vi "funnels to Commands.vi"(1 "funnels":T7(array[cluster]), 2 "Funnel Properties":T3[](array[typedef])=[{"Enabled"=TRUE, "Direction"=0, "Smooth Segments"=12.0, "Bottom Segs."=20.0, "Speed (um/s)"={"Schedule"=enum."Constant", "Settings"=variant(dbl 0.0)}, "Voltage (V)"={"Schedule"=enum."Constant", "Settings"=variant(dbl 0.0)}, "Set Resistance"=enum."1G ohm"}, {"Enabled"=TRUE, "Direction"=0, "Smooth Segments"=12.0, "Bottom Segs."=20.0, "Speed (um/s)"={"Schedule"=enum."Constant", "Settings"=variant(dbl 0.0)}, "Voltage (V)"={"Schedule"=enum."Constant", "Settings"=variant(dbl 0.0)}, "Set Resistance"=enum."1G ohm"}, {"Enabled"=TRUE, "Direction"=0, "Smooth Segments"=12.0, "Bottom Segs."=20.0, "Speed (um/s)"={"Schedule"=enum."Constant", "Settings"=variant(dbl 0.0)}, "Voltage (V)"={"Schedule"=enum."Constant", "Settings"=variant(dbl 0.0)}, "Set Resistance"=enum."1G ohm"}, {"Enabled"=TRUE, "Direction"=0, "Smooth Segments"=12.0, "Bottom Segs."=20.0, "Speed (um/s)"={"Schedule"=enum."Constant", "Settings"=variant(dbl 0.0)}, "Voltage (V)"={"Schedule"=enum."Constant", "Settings"=variant(dbl 0.0)}, "Set Resistance"=enum."1G ohm"}, {"Enabled"=TRUE, "Direction"=0, "Smooth Segments"=12.0, "Bottom Segs."=20.0, "Speed (um/s)"={"Schedule"=enum."Constant", "Settings"=variant(dbl 0.0)}, "Voltage (V)"={"Schedule"=enum."Constant", "Settings"=variant(dbl 0.0)}, "Set Resistance"=enum."1G ohm"}, {"Enabled"=TRUE, "Direction"=0, "Smooth Segments"=12.0, "Bottom Segs."=20.0, "Speed (um/s)"={"Schedule"=enum."Constant", "Settings"=variant(dbl 0.0)}, "Voltage (V)"={"Schedule"=enum."Constant", "Settings"=variant(dbl 0.0)}, "Set Resistance"=enum."1G ohm"}, {"Enabled"=TRUE, "Direction"=0, "Smooth Segments"=12.0, "Bottom Segs."=20.0, "Speed (um/s)"={"Schedule"=enum."Constant", "Settings"=variant(dbl 0.0)}, "Voltage (V)"={"Schedule"=enum."Constant", "Settings"=variant(dbl 0.0)}, "Set Resistance"=enum."1G ohm"}, {"Enabled"=TRUE, "Direction"=0, "Smooth Segments"=12.0, "Bottom Segs."=20.0, "Speed (um/s)"={"Schedule"=enum."Constant", "Settings"=variant(dbl 0.0)}, "Voltage (V)"={"Schedule"=enum."Constant", "Settings"=variant(dbl 0.0)}, "Set Resistance"=enum."1G ohm"}, {"Enabled"=TRUE, "Direction"=0, "Smooth Segments"=12.0, "Bottom Segs."=20.0, "Speed (um/s)"={"Schedule"=enum."Constant", "Settings"=variant(dbl 0.0)}, "Voltage (V)"={"Schedule"=enum."Constant", "Settings"=variant(dbl 0.0)}, "Set Resistance"=enum."1G ohm"}, {"Enabled"=TRUE, "Direction"=0, "Smooth Segments"=12.0, "Bottom Segs."=20.0, "Speed (um/s)"={"Schedule"=enum."Constant", "Settings"=variant(dbl 0.0)}, "Voltage (V)"={"Schedule"=enum."Constant", "Settings"=variant(dbl 0.0)}, "Set Resistance"=enum."1G ohm"}, {"Enabled"=TRUE, "Direction"=0, "Smooth Segments"=12.0, "Bottom Segs."=20.0, "Speed (um/s)"={"Schedule"=enum."Constant", "Settings"=variant(dbl 0.0)}, "Voltage (V)"={"Schedule"=enum."Constant", "Settings"=variant(dbl 0.0)}, "Set Resistance"=enum."1G ohm"}, {"Enabled"=TRUE, "Direction"=0, "Smooth Segments"=12.0, "Bottom Segs."=20.0, "Speed (um/s)"={"Schedule"=enum."Constant", "Settings"=variant(dbl 0.0)}, "Voltage (V)"={"Schedule"=enum."Constant", "Settings"=variant(dbl 0.0)}, "Set Resistance"=enum."1G ohm"}, {"Enabled"=TRUE, "Direction"=0, "Smooth Segments"=12.0, "Bottom Segs."=20.0, "Speed (um/s)"={"Schedule"=enum."Constant", "Settings"=variant(dbl 0.0)}, "Voltage (V)"={"Schedule"=enum."Constant", "Settings"=variant(dbl 0.0)}, "Set Resistance"=enum."1G ohm"}, {"Enabled"=TRUE, "Direction"=0, "Smooth Segments"=12.0, "Bottom Segs."=20.0, "Speed (um/s)"={"Schedule"=enum."Constant", "Settings"=variant(dbl 0.0)}, "Voltage (V)"={"Schedule"=enum."Constant", "Settings"=variant(dbl 0.0)}, "Set Resistance"=enum."1G ohm"}, {"Enabled"=TRUE, "Direction"=0, "Smooth Segments"=12.0, "Bottom Segs."=20.0, "Speed (um/s)"={"Schedule"=enum."Constant", "Settings"=variant(dbl 0.0)}, "Voltage (V)"={"Schedule"=enum."Constant", "Settings"=variant(dbl 0.0)}, "Set Resistance"=enum."1G ohm"}, {"Enabled"=TRUE, "Direction"=0, "Smooth Segments"=12.0, "Bottom Segs."=20.0, "Speed (um/s)"={"Schedule"=enum."Constant", "Settings"=variant(dbl 0.0)}, "Voltage (V)"={"Schedule"=enum."Constant", "Settings"=variant(dbl 0.0)}, "Set Resistance"=enum."1G ohm"}, {"Enabled"=TRUE, "Direction"=0, "Smooth Segments"=12.0, "Bottom Segs."=20.0, "Speed (um/s)"={"Schedule"=enum."Constant", "Settings"=variant(dbl 0.0)}, "Voltage (V)"={"Schedule"=enum."Constant", "Settings"=variant(dbl 0.0)}, "Set Resistance"=enum."1G ohm"}, {"Enabled"=TRUE, "Direction"=0, "Smooth Segments"=12.0, "Bottom Segs."=20.0, "Speed (um/s)"={"Schedule"=enum."Constant", "Settings"=variant(dbl 0.0)}, "Voltage (V)"={"Schedule"=enum."Constant", "Settings"=variant(dbl 0.0)}, "Set Resistance"=enum."1G ohm"}, {"Enabled"=TRUE, "Direction"=0, "Smooth Segments"=12.0, "Bottom Segs."=20.0, "Speed (um/s)"={"Schedule"=enum."Constant", "Settings"=variant(dbl 0.0)}, "Voltage (V)"={"Schedule"=enum."Constant", "Settings"=variant(dbl 0.0)}, "Set Resistance"=enum."1G ohm"}, {"Enabled"=TRUE, "Direction"=0, "Smooth Segments"=12.0, "Bottom Segs."=20.0, "Speed (um/s)"={"Schedule"=enum."Constant", "Settings"=variant(dbl 0.0)}, "Voltage (V)"={"Schedule"=enum."Constant", "Settings"=variant(dbl 0.0)}, "Set Resistance"=enum."1G ohm"}, {"Enabled"=TRUE, "Direction"=0, "Smooth Segments"=12.0, "Bottom Segs."=20.0, "Speed (um/s)"={"Schedule"=enum."Constant", "Settings"=variant(dbl 0.0)}, "Voltage (V)"={"Schedule"=enum."Constant", "Settings"=variant(dbl 0.0)}, "Set Resistance"=enum."1G ohm"}, {"Enabled"=TRUE, "Direction"=0, "Smooth Segments"=12.0, "Bottom Segs."=20.0, "Speed (um/s)"={"Schedule"=enum."Constant", "Settings"=variant(dbl 0.0)}, "Voltage (V)"={"Schedule"=enum."Constant", "Settings"=variant(dbl 0.0)}, "Set Resistance"=enum."1G ohm"}, {"Enabled"=TRUE, "Direction"=0, "Smooth Segments"=12.0, "Bottom Segs."=20.0, "Speed (um/s)"={"Schedule"=enum."Constant", "Settings"=variant(dbl 0.0)}, "Voltage (V)"={"Schedule"=enum."Constant", "Settings"=variant(dbl 0.0)}, "Set Resistance"=enum."1G ohm"}, {"Enabled"=TRUE, "Direction"=0, "Smooth Segments"=12.0, "Bottom Segs."=20.0, "Speed (um/s)"={"Schedule"=enum."Constant", "Settings"=variant(dbl 0.0)}, "Voltage (V)"={"Schedule"=enum."Constant", "Settings"=variant(dbl 0.0)}, "Set Resistance"=enum."1G ohm"}, {"Enabled"=TRUE, "Direction"=0, "Smooth Segments"=12.0, "Bottom Segs."=20.0, "Speed (um/s)"={"Schedule"=enum."Constant", "Settings"=variant(dbl 0.0)}, "Voltage (V)"={"Schedule"=enum."Constant", "Settings"=variant(dbl 0.0)}, "Set Resistance"=enum."1G ohm"}, {"Enabled"=TRUE, "Direction"=0, "Smooth Segments"=12.0, "Bottom Segs."=20.0, "Speed (um/s)"={"Schedule"=enum."Constant", "Settings"=variant(dbl 0.0)}, "Voltage (V)"={"Schedule"=enum."Constant", "Settings"=variant(dbl 0.0)}, "Set Resistance"=enum."1G ohm"}, {"Enabled"=TRUE, "Direction"=0, "Smooth Segments"=12.0, "Bottom Segs."=20.0, "Speed (um/s)"={"Schedule"=enum."Constant", "Settings"=variant(dbl 0.0)}, "Voltage (V)"={"Schedule"=enum."Constant", "Settings"=variant(dbl 0.0)}, "Set Resistance"=enum."1G ohm"}, {"Enabled"=TRUE, "Direction"=0, "Smooth Segments"=12.0, "Bottom Segs."=20.0, "Speed (um/s)"={"Schedule"=enum."Constant", "Settings"=variant(dbl 0.0)}, "Voltage (V)"={"Schedule"=enum."Constant", "Settings"=variant(dbl 0.0)}, "Set Resistance"=enum."1G ohm"}, {"Enabled"=TRUE, "Direction"=0, "Smooth Segments"=12.0, "Bottom Segs."=20.0, "Speed (um/s)"={"Schedule"=enum."Constant", "Settings"=variant(dbl 0.0)}, "Voltage (V)"={"Schedule"=enum."Constant", "Settings"=variant(dbl 0.0)}, "Set Resistance"=enum."1G ohm"}, {"Enabled"=TRUE, "Direction"=0, "Smooth Segments"=12.0, "Bottom Segs."=20.0, "Speed (um/s)"={"Schedule"=enum."Constant", "Settings"=variant(dbl 0.0)}, "Voltage (V)"={"Schedule"=enum."Constant", "Settings"=variant(dbl 0.0)}, "Set Resistance"=enum."1G ohm"}, {"Enabled"=TRUE, "Direction"=0, "Smooth Segments"=12.0, "Bottom Segs."=20.0, "Speed (um/s)"={"Schedule"=enum."Constant", "Settings"=variant(dbl 0.0)}, "Voltage (V)"={"Schedule"=enum."Constant", "Settings"=variant(dbl 0.0)}, "Set Resistance"=enum."1G ohm"}, {"Enabled"=TRUE, "Direction"=0, "Smooth Segments"=12.0, "Bottom Segs."=20.0, "Speed (um/s)"={"Schedule"=enum."Constant", "Settings"=variant(dbl 0.0)}, "Voltage (V)"={"Schedule"=enum."Constant", "Settings"=variant(dbl 0.0)}, "Set Resistance"=enum."1G ohm"}, {"Enabled"=TRUE, "Direction"=0, "Smooth Segments"=12.0, "Bottom Segs."=20.0, "Speed (um/s)"={"Schedule"=enum."Constant", "Settings"=variant(dbl 0.0)}, "Voltage (V)"={"Schedule"=enum."Constant", "Settings"=variant(dbl 0.0)}, "Set Resistance"=enum."1G ohm"}, {"Enabled"=TRUE, "Direction"=0, "Smooth Segments"=12.0, "Bottom Segs."=20.0, "Speed (um/s)"={"Schedule"=enum."Constant", "Settings"=variant(dbl 0.0)}, "Voltage (V)"={"Schedule"=enum."Constant", "Settings"=variant(dbl 0.0)}, "Set Resistance"=enum."1G ohm"}, {"Enabled"=TRUE, "Direction"=0, "Smooth Segments"=12.0, "Bottom Segs."=20.0, "Speed (um/s)"={"Schedule"=enum."Constant", "Settings"=variant(dbl 0.0)}, "Voltage (V)"={"Schedule"=enum."Constant", "Settings"=variant(dbl 0.0)}, "Set Resistance"=enum."1G ohm"}, {"Enabled"=TRUE, "Direction"=0, "Smooth Segments"=12.0, "Bottom Segs."=20.0, "Speed (um/s)"={"Schedule"=enum."Constant", "Settings"=variant(dbl 0.0)}, "Voltage (V)"={"Schedule"=enum."Constant", "Settings"=variant(dbl 0.0)}, "Set Resistance"=enum."1G ohm"}, {"Enabled"=TRUE, "Direction"=0, "Smooth Segments"=12.0, "Bottom Segs."=20.0, "Speed (um/s)"={"Schedule"=enum."Constant", "Settings"=variant(dbl 0.0)}, "Voltage (V)"={"Schedule"=enum."Constant", "Settings"=variant(dbl 0.0)}, "Set Resistance"=enum."1G ohm"}, {"Enabled"=TRUE, "Direction"=0, "Smooth Segments"=12.0, "Bottom Segs."=20.0, "Speed (um/s)"={"Schedule"=enum."Constant", "Settings"=variant(dbl 0.0)}, "Voltage (V)"={"Schedule"=enum."Constant", "Settings"=variant(dbl 0.0)}, "Set Resistance"=enum."1G ohm"}, {"Enabled"=TRUE, "Direction"=0, "Smooth Segments"=12.0, "Bottom Segs."=20.0, "Speed (um/s)"={"Schedule"=enum."Constant", "Settings"=variant(dbl 0.0)}, "Voltage (V)"={"Schedule"=enum."Constant", "Settings"=variant(dbl 0.0)}, "Set Resistance"=enum."1G ohm"}, {"Enabled"=TRUE, "Direction"=0, "Smooth Segments"=12.0, "Bottom Segs."=20.0, "Speed (um/s)"={"Schedule"=enum."Constant", "Settings"=variant(dbl 0.0)}, "Voltage (V)"={"Schedule"=enum."Constant", "Settings"=variant(dbl 0.0)}, "Set Resistance"=enum."1G ohm"}, {"Enabled"=TRUE, "Direction"=0, "Smooth Segments"=12.0, "Bottom Segs."=20.0, "Speed (um/s)"={"Schedule"=enum."Constant", "Settings"=variant(dbl 0.0)}, "Voltage (V)"={"Schedule"=enum."Constant", "Settings"=variant(dbl 0.0)}, "Set Resistance"=enum."1G ohm"}, {"Enabled"=TRUE, "Direction"=0, "Smooth Segments"=12.0, "Bottom Segs."=20.0, "Speed (um/s)"={"Schedule"=enum."Constant", "Settings"=variant(dbl 0.0)}, "Voltage (V)"={"Schedule"=enum."Constant", "Settings"=variant(dbl 0.0)}, "Set Resistance"=enum."1G ohm"}, {"Enabled"=TRUE, "Direction"=0, "Smooth Segments"=12.0, "Bottom Segs."=20.0, "Speed (um/s)"={"Schedule"=enum."Constant", "Settings"=variant(dbl 0.0)}, "Voltage (V)"={"Schedule"=enum."Constant", "Settings"=variant(dbl 0.0)}, "Set Resistance"=enum."1G ohm"}, {"Enabled"=TRUE, "Direction"=0, "Smooth Segments"=12.0, "Bottom Segs."=20.0, "Speed (um/s)"={"Schedule"=enum."Constant", "Settings"=variant(dbl 0.0)}, "Voltage (V)"={"Schedule"=enum."Constant", "Settings"=variant(dbl 0.0)}, "Set Resistance"=enum."1G ohm"}, {"Enabled"=TRUE, "Direction"=0, "Smooth Segments"=12.0, "Bottom Segs."=20.0, "Speed (um/s)"={"Schedule"=enum."Constant", "Settings"=variant(dbl 0.0)}, "Voltage (V)"={"Schedule"=enum."Constant", "Settings"=variant(dbl 0.0)}, "Set Resistance"=enum."1G ohm"}, {"Enabled"=TRUE, "Direction"=0, "Smooth Segments"=12.0, "Bottom Segs."=20.0, "Speed (um/s)"={"Schedule"=enum."Constant", "Settings"=variant(dbl 0.0)}, "Voltage (V)"={"Schedule"=enum."Constant", "Settings"=variant(dbl 0.0)}, "Set Resistance"=enum."1G ohm"}, {"Enabled"=TRUE, "Direction"=0, "Smooth Segments"=12.0, "Bottom Segs."=20.0, "Speed (um/s)"={"Schedule"=enum."Constant", "Settings"=variant(dbl 0.0)}, "Voltage (V)"={"Schedule"=enum."Constant", "Settings"=variant(dbl 0.0)}, "Set Resistance"=enum."1G ohm"}, {"Enabled"=TRUE, "Direction"=0, "Smooth Segments"=12.0, "Bottom Segs."=20.0, "Speed (um/s)"={"Schedule"=enum."Constant", "Settings"=variant(dbl 0.0)}, "Voltage (V)"={"Schedule"=enum."Constant", "Settings"=variant(dbl 0.0)}, "Set Resistance"=enum."1G ohm"}, {"Enabled"=TRUE, "Direction"=0, "Smooth Segments"=12.0, "Bottom Segs."=20.0, "Speed (um/s)"={"Schedule"=enum."Constant", "Settings"=variant(dbl 0.0)}, "Voltage (V)"={"Schedule"=enum."Constant", "Settings"=variant(dbl 0.0)}, "Set Resistance"=enum."1G ohm"}, {"Enabled"=TRUE, "Direction"=0, "Smooth Segments"=12.0, "Bottom Segs."=20.0, "Speed (um/s)"={"Schedule"=enum."Constant", "Settings"=variant(dbl 0.0)}, "Voltage (V)"={"Schedule"=enum."Constant", "Settings"=variant(dbl 0.0)}, "Set Resistance"=enum."1G ohm"}, {"Enabled"=TRUE, "Direction"=0, "Smooth Segments"=12.0, "Bottom Segs."=20.0, "Speed (um/s)"={"Schedule"=enum."Constant", "Settings"=variant(dbl 0.0)}, "Voltage (V)"={"Schedule"=enum."Constant", "Settings"=variant(dbl 0.0)}, "Set Resistance"=enum."1G ohm"}, {"Enabled"=TRUE, "Direction"=0, "Smooth Segments"=12.0, "Bottom Segs."=20.0, "Speed (um/s)"={"Schedule"=enum."Constant", "Settings"=variant(dbl 0.0)}, "Voltage (V)"={"Schedule"=enum."Constant", "Settings"=variant(dbl 0.0)}, "Set Resistance"=enum."1G ohm"}, {"Enabled"=TRUE, "Direction"=0, "Smooth Segments"=12.0, "Bottom Segs."=20.0, "Speed (um/s)"={"Schedule"=enum."Constant", "Settings"=variant(dbl 0.0)}, "Voltage (V)"={"Schedule"=enum."Constant", "Settings"=variant(dbl 0.0)}, "Set Resistance"=enum."1G ohm"}, {"Enabled"=TRUE, "Direction"=0, "Smooth Segments"=12.0, "Bottom Segs."=20.0, "Speed (um/s)"={"Schedule"=enum."Constant", "Settings"=variant(dbl 0.0)}, "Voltage (V)"={"Schedule"=enum."Constant", "Settings"=variant(dbl 0.0)}, "Set Resistance"=enum."1G ohm"}, {"Enabled"=TRUE, "Direction"=0, "Smooth Segments"=12.0, "Bottom Segs."=20.0, "Speed (um/s)"={"Schedule"=enum."Constant", "Settings"=variant(dbl 0.0)}, "Voltage (V)"={"Schedule"=enum."Constant", "Settings"=variant(dbl 0.0)}, "Set Resistance"=enum."1G ohm"}, {"Enabled"=TRUE, "Direction"=0, "Smooth Segments"=12.0, "Bottom Segs."=20.0, "Speed (um/s)"={"Schedule"=enum."Constant", "Settings"=variant(dbl 0.0)}, "Voltage (V)"={"Schedule"=enum."Constant", "Settings"=variant(dbl 0.0)}, "Set Resistance"=enum."1G ohm"}, {"Enabled"=TRUE, "Direction"=0, "Smooth Segments"=12.0, "Bottom Segs."=20.0, "Speed (um/s)"={"Schedule"=enum."Constant", "Settings"=variant(dbl 0.0)}, "Voltage (V)"={"Schedule"=enum."Constant", "Settings"=variant(dbl 0.0)}, "Set Resistance"=enum."1G ohm"}, {"Enabled"=TRUE, "Direction"=0, "Smooth Segments"=12.0, "Bottom Segs."=20.0, "Speed (um/s)"={"Schedule"=enum."Constant", "Settings"=variant(dbl 0.0)}, "Voltage (V)"={"Schedule"=enum."Constant", "Settings"=variant(dbl 0.0)}, "Set Resistance"=enum."1G ohm"}, {"Enabled"=TRUE, "Direction"=0, "Smooth Segments"=12.0, "Bottom Segs."=20.0, "Speed (um/s)"={"Schedule"=enum."Constant", "Settings"=variant(dbl 0.0)}, "Voltage (V)"={"Schedule"=enum."Constant", "Settings"=variant(dbl 0.0)}, "Set Resistance"=enum."1G ohm"}, {"Enabled"=TRUE, "Direction"=0, "Smooth Segments"=12.0, "Bottom Segs."=20.0, "Speed (um/s)"={"Schedule"=enum."Constant", "Settings"=variant(dbl 0.0)}, "Voltage (V)"={"Schedule"=enum."Constant", "Settings"=variant(dbl 0.0)}, "Set Resistance"=enum."1G ohm"}, {"Enabled"=TRUE, "Direction"=0, "Smooth Segments"=12.0, "Bottom Segs."=20.0, "Speed (um/s)"={"Schedule"=enum."Constant", "Settings"=variant(dbl 0.0)}, "Voltage (V)"={"Schedule"=enum."Constant", "Settings"=variant(dbl 0.0)}, "Set Resistance"=enum."1G ohm"}, {"Enabled"=TRUE, "Direction"=0, "Smooth Segments"=12.0, "Bottom Segs."=20.0, "Speed (um/s)"={"Schedule"=enum."Constant", "Settings"=variant(dbl 0.0)}, "Voltage (V)"={"Schedule"=enum."Constant", "Settings"=variant(dbl 0.0)}, "Set Resistance"=enum."1G ohm"}, {"Enabled"=TRUE, "Direction"=0, "Smooth Segments"=12.0, "Bottom Segs."=20.0, "Speed (um/s)"={"Schedule"=enum."Constant", "Settings"=variant(dbl 0.0)}, "Voltage (V)"={"Schedule"=enum."Constant", "Settings"=variant(dbl 0.0)}, "Set Resistance"=enum."1G ohm"}, {"Enabled"=TRUE, "Direction"=0, "Smooth Segments"=12.0, "Bottom Segs."=20.0, "Speed (um/s)"={"Schedule"=enum."Constant", "Settings"=variant(dbl 0.0)}, "Voltage (V)"={"Schedule"=enum."Constant", "Settings"=variant(dbl 0.0)}, "Set Resistance"=enum."1G ohm"}, {"Enabled"=TRUE, "Direction"=0, "Smooth Segments"=12.0, "Bottom Segs."=20.0, "Speed (um/s)"={"Schedule"=enum."Constant", "Settings"=variant(dbl 0.0)}, "Voltage (V)"={"Schedule"=enum."Constant", "Settings"=variant(dbl 0.0)}, "Set Resistance"=enum."1G ohm"}, {"Enabled"=TRUE, "Direction"=0, "Smooth Segments"=12.0, "Bottom Segs."=20.0, "Speed (um/s)"={"Schedule"=enum."Constant", "Settings"=variant(dbl 0.0)}, "Voltage (V)"={"Schedule"=enum."Constant", "Settings"=variant(dbl 0.0)}, "Set Resistance"=enum."1G ohm"}, {"Enabled"=TRUE, "Direction"=0, "Smooth Segments"=12.0, "Bottom Segs."=20.0, "Speed (um/s)"={"Schedule"=enum."Constant", "Settings"=variant(dbl 0.0)}, "Voltage (V)"={"Schedule"=enum."Constant", "Settings"=variant(dbl 0.0)}, "Set Resistance"=enum."1G ohm"}, {"Enabled"=TRUE, "Direction"=0, "Smooth Segments"=12.0, "Bottom Segs."=20.0, "Speed (um/s)"={"Schedule"=enum."Constant", "Settings"=variant(dbl 0.0)}, "Voltage (V)"={"Schedule"=enum."Constant", "Settings"=variant(dbl 0.0)}, "Set Resistance"=enum."1G ohm"}, {"Enabled"=TRUE, "Direction"=0, "Smooth Segments"=12.0, "Bottom Segs."=20.0, "Speed (um/s)"={"Schedule"=enum."Constant", "Settings"=variant(dbl 0.0)}, "Voltage (V)"={"Schedule"=enum."Constant", "Settings"=variant(dbl 0.0)}, "Set Resistance"=enum."1G ohm"}, {"Enabled"=TRUE, "Direction"=0, "Smooth Segments"=12.0, "Bottom Segs."=20.0, "Speed (um/s)"={"Schedule"=enum."Constant", "Settings"=variant(dbl 0.0)}, "Voltage (V)"={"Schedule"=enum."Constant", "Settings"=variant(dbl 0.0)}, "Set Resistance"=enum."1G ohm"}, {"Enabled"=TRUE, "Direction"=0, "Smooth Segments"=12.0, "Bottom Segs."=20.0, "Speed (um/s)"={"Schedule"=enum."Constant", "Settings"=variant(dbl 0.0)}, "Voltage (V)"={"Schedule"=enum."Constant", "Settings"=variant(dbl 0.0)}, "Set Resistance"=enum."1G ohm"}, {"Enabled"=TRUE, "Direction"=0, "Smooth Segments"=12.0, "Bottom Segs."=20.0, "Speed (um/s)"={"Schedule"=enum."Constant", "Settings"=variant(dbl 0.0)}, "Voltage (V)"={"Schedule"=enum."Constant", "Settings"=variant(dbl 0.0)}, "Set Resistance"=enum."1G ohm"}, {"Enabled"=TRUE, "Direction"=0, "Smooth Segments"=12.0, "Bottom Segs."=20.0, "Speed (um/s)"={"Schedule"=enum."Constant", "Settings"=variant(dbl 0.0)}, "Voltage (V)"={"Schedule"=enum."Constant", "Settings"=variant(dbl 0.0)}, "Set Resistance"=enum."1G ohm"}, {"Enabled"=TRUE, "Direction"=0, "Smooth Segments"=12.0, "Bottom Segs."=20.0, "Speed (um/s)"={"Schedule"=enum."Constant", "Settings"=variant(dbl 0.0)}, "Voltage (V)"={"Schedule"=enum."Constant", "Settings"=variant(dbl 0.0)}, "Set Resistance"=enum."1G ohm"}, {"Enabled"=TRUE, "Direction"=0, "Smooth Segments"=12.0, "Bottom Segs."=20.0, "Speed (um/s)"={"Schedule"=enum."Constant", "Settings"=variant(dbl 0.0)}, "Voltage (V)"={"Schedule"=enum."Constant", "Settings"=variant(dbl 0.0)}, "Set Resistance"=enum."1G ohm"}, {"Enabled"=TRUE, "Direction"=0, "Smooth Segments"=12.0, "Bottom Segs."=20.0, "Speed (um/s)"={"Schedule"=enum."Constant", "Settings"=variant(dbl 0.0)}, "Voltage (V)"={"Schedule"=enum."Constant", "Settings"=variant(dbl 0.0)}, "Set Resistance"=enum."1G ohm"}, {"Enabled"=TRUE, "Direction"=0, "Smooth Segments"=12.0, "Bottom Segs."=20.0, "Speed (um/s)"={"Schedule"=enum."Constant", "Settings"=variant(dbl 0.0)}, "Voltage (V)"={"Schedule"=enum."Constant", "Settings"=variant(dbl 0.0)}, "Set Resistance"=enum."1G ohm"}, {"Enabled"=TRUE, "Direction"=0, "Smooth Segments"=12.0, "Bottom Segs."=20.0, "Speed (um/s)"={"Schedule"=enum."Constant", "Settings"=variant(dbl 0.0)}, "Voltage (V)"={"Schedule"=enum."Constant", "Settings"=variant(dbl 0.0)}, "Set Resistance"=enum."1G ohm"}, {"Enabled"=TRUE, "Direction"=0, "Smooth Segments"=12.0, "Bottom Segs."=20.0, "Speed (um/s)"={"Schedule"=enum."Constant", "Settings"=variant(dbl 0.0)}, "Voltage (V)"={"Schedule"=enum."Constant", "Settings"=variant(dbl 0.0)}, "Set Resistance"=enum."1G ohm"}, {"Enabled"=TRUE, "Direction"=0, "Smooth Segments"=12.0, "Bottom Segs."=20.0, "Speed (um/s)"={"Schedule"=enum."Constant", "Settings"=variant(dbl 0.0)}, "Voltage (V)"={"Schedule"=enum."Constant", "Settings"=variant(dbl 0.0)}, "Set Resistance"=enum."1G ohm"}, {"Enabled"=TRUE, "Direction"=0, "Smooth Segments"=12.0, "Bottom Segs."=20.0, "Speed (um/s)"={"Schedule"=enum."Constant", "Settings"=variant(dbl 0.0)}, "Voltage (V)"={"Schedule"=enum."Constant", "Settings"=variant(dbl 0.0)}, "Set Resistance"=enum."1G ohm"}, {"Enabled"=TRUE, "Direction"=0, "Smooth Segments"=12.0, "Bottom Segs."=20.0, "Speed (um/s)"={"Schedule"=enum."Constant", "Settings"=variant(dbl 0.0)}, "Voltage (V)"={"Schedule"=enum."Constant", "Settings"=variant(dbl 0.0)}, "Set Resistance"=enum."1G ohm"}, {"Enabled"=TRUE, "Direction"=0, "Smooth Segments"=12.0, "Bottom Segs."=20.0, "Speed (um/s)"={"Schedule"=enum."Constant", "Settings"=variant(dbl 0.0)}, "Voltage (V)"={"Schedule"=enum."Constant", "Settings"=variant(dbl 0.0)}, "Set Resistance"=enum."1G ohm"}, {"Enabled"=TRUE, "Direction"=0, "Smooth Segments"=12.0, "Bottom Segs."=20.0, "Speed (um/s)"={"Schedule"=enum."Constant", "Settings"=variant(dbl 0.0)}, "Voltage (V)"={"Schedule"=enum."Constant", "Settings"=variant(dbl 0.0)}, "Set Resistance"=enum."1G ohm"}, {"Enabled"=TRUE, "Direction"=0, "Smooth Segments"=12.0, "Bottom Segs."=20.0, "Speed (um/s)"={"Schedule"=enum."Constant", "Settings"=variant(dbl 0.0)}, "Voltage (V)"={"Schedule"=enum."Constant", "Settings"=variant(dbl 0.0)}, "Set Resistance"=enum."1G ohm"}, {"Enabled"=TRUE, "Direction"=0, "Smooth Segments"=12.0, "Bottom Segs."=20.0, "Speed (um/s)"={"Schedule"=enum."Constant", "Settings"=variant(dbl 0.0)}, "Voltage (V)"={"Schedule"=enum."Constant", "Settings"=variant(dbl 0.0)}, "Set Resistance"=enum."1G ohm"}, {"Enabled"=TRUE, "Direction"=0, "Smooth Segments"=12.0, "Bottom Segs."=20.0, "Speed (um/s)"={"Schedule"=enum."Constant", "Settings"=variant(dbl 0.0)}, "Voltage (V)"={"Schedule"=enum."Constant", "Settings"=variant(dbl 0.0)}, "Set Resistance"=enum."1G ohm"}, {"Enabled"=TRUE, "Direction"=0, "Smooth Segments"=12.0, "Bottom Segs."=20.0, "Speed (um/s)"={"Schedule"=enum."Constant", "Settings"=variant(dbl 0.0)}, "Voltage (V)"={"Schedule"=enum."Constant", "Settings"=variant(dbl 0.0)}, "Set Resistance"=enum."1G ohm"}, {"Enabled"=TRUE, "Direction"=0, "Smooth Segments"=12.0, "Bottom Segs."=20.0, "Speed (um/s)"={"Schedule"=enum."Constant", "Settings"=variant(dbl 0.0)}, "Voltage (V)"={"Schedule"=enum."Constant", "Settings"=variant(dbl 0.0)}, "Set Resistance"=enum."1G ohm"}, {"Enabled"=TRUE, "Direction"=0, "Smooth Segments"=12.0, "Bottom Segs."=20.0, "Speed (um/s)"={"Schedule"=enum."Constant", "Settings"=variant(dbl 0.0)}, "Voltage (V)"={"Schedule"=enum."Constant", "Settings"=variant(dbl 0.0)}, "Set Resistance"=enum."1G ohm"}, {"Enabled"=TRUE, "Direction"=0, "Smooth Segments"=12.0, "Bottom Segs."=20.0, "Speed (um/s)"={"Schedule"=enum."Constant", "Settings"=variant(dbl 0.0)}, "Voltage (V)"={"Schedule"=enum."Constant", "Settings"=variant(dbl 0.0)}, "Set Resistance"=enum."1G ohm"}, {"Enabled"=TRUE, "Direction"=0, "Smooth Segments"=12.0, "Bottom Segs."=20.0, "Speed (um/s)"={"Schedule"=enum."Constant", "Settings"=variant(dbl 0.0)}, "Voltage (V)"={"Schedule"=enum."Constant", "Settings"=variant(dbl 0.0)}, "Set Resistance"=enum."1G ohm"}, {"Enabled"=TRUE, "Direction"=0, "Smooth Segments"=12.0, "Bottom Segs."=20.0, "Speed (um/s)"={"Schedule"=enum."Constant", "Settings"=variant(dbl 0.0)}, "Voltage (V)"={"Schedule"=enum."Constant", "Settings"=variant(dbl 0.0)}, "Set Resistance"=enum."1G ohm"}, {"Enabled"=TRUE, "Direction"=0, "Smooth Segments"=12.0, "Bottom Segs."=20.0, "Speed (um/s)"={"Schedule"=enum."Constant", "Settings"=variant(dbl 0.0)}, "Voltage (V)"={"Schedule"=enum."Constant", "Settings"=variant(dbl 0.0)}, "Set Resistance"=enum."1G ohm"}, {"Enabled"=TRUE, "Direction"=0, "Smooth Segments"=12.0, "Bottom Segs."=20.0, "Speed (um/s)"={"Schedule"=enum."Constant", "Settings"=variant(dbl 0.0)}, "Voltage (V)"={"Schedule"=enum."Constant", "Settings"=variant(dbl 0.0)}, "Set Resistance"=enum."1G ohm"}, {"Enabled"=TRUE, "Direction"=0, "Smooth Segments"=12.0, "Bottom Segs."=20.0, "Speed (um/s)"={"Schedule"=enum."Constant", "Settings"=variant(dbl 0.0)}, "Voltage (V)"={"Schedule"=enum."Constant", "Settings"=variant(dbl 0.0)}, "Set Resistance"=enum."1G ohm"}, {"Enabled"=TRUE, "Direction"=0, "Smooth Segments"=12.0, "Bottom Segs."=20.0, "Speed (um/s)"={"Schedule"=enum."Constant", "Settings"=variant(dbl 0.0)}, "Voltage (V)"={"Schedule"=enum."Constant", "Settings"=variant(dbl 0.0)}, "Set Resistance"=enum."1G ohm"}, {"Enabled"=TRUE, "Direction"=0, "Smooth Segments"=12.0, "Bottom Segs."=20.0, "Speed (um/s)"={"Schedule"=enum."Constant", "Settings"=variant(dbl 0.0)}, "Voltage (V)"={"Schedule"=enum."Constant", "Settings"=variant(dbl 0.0)}, "Set Resistance"=enum."1G ohm"}, {"Enabled"=TRUE, "Direction"=0, "Smooth Segments"=12.0, "Bottom Segs."=20.0, "Speed (um/s)"={"Schedule"=enum."Constant", "Settings"=variant(dbl 0.0)}, "Voltage (V)"={"Schedule"=enum."Constant", "Settings"=variant(dbl 0.0)}, "Set Resistance"=enum."1G ohm"}, {"Enabled"=TRUE, "Direction"=0, "Smooth Segments"=12.0, "Bottom Segs."=20.0, "Speed (um/s)"={"Schedule"=enum."Constant", "Settings"=variant(dbl 0.0)}, "Voltage (V)"={"Schedule"=enum."Constant", "Settings"=variant(dbl 0.0)}, "Set Resistance"=enum."1G ohm"}, {"Enabled"=TRUE, "Direction"=0, "Smooth Segments"=12.0, "Bottom Segs."=20.0, "Speed (um/s)"={"Schedule"=enum."Constant", "Settings"=variant(dbl 0.0)}, "Voltage (V)"={"Schedule"=enum."Constant", "Settings"=variant(dbl 0.0)}, "Set Resistance"=enum."1G ohm"}] {"Direction" items=["Forward", "Backward"]}) -> (0 "Lithography Data":T2(array[cluster]))   [LabVIEW 2019]
doc: "This VI processes the rectangles' data and outputs lithography data."
uses:
  <vilib>/Analysis/Matrix/Datatypes/RealMatrix.ctl
  typedefs/Funnel Properties - cluster.ctl
  typedefs/Voltage - cluster.ctl
  typedefs/Schedule - enum.ctl
  <userlib>/LevyLab/Relay Box/Typedefs/Resistor--enum.ctl
  <userlib>/_OpenG.lib/array/array.llb/Search 1D Array (String)__ogtk.vi
  <userlib>/LevyLab/Relay Box/Relay-Box.lvclass
  <vilib>/Analysis/Matrix/NI_Matrix.lvlib
panel:
  # "MONSTER CLUSTER!!!"
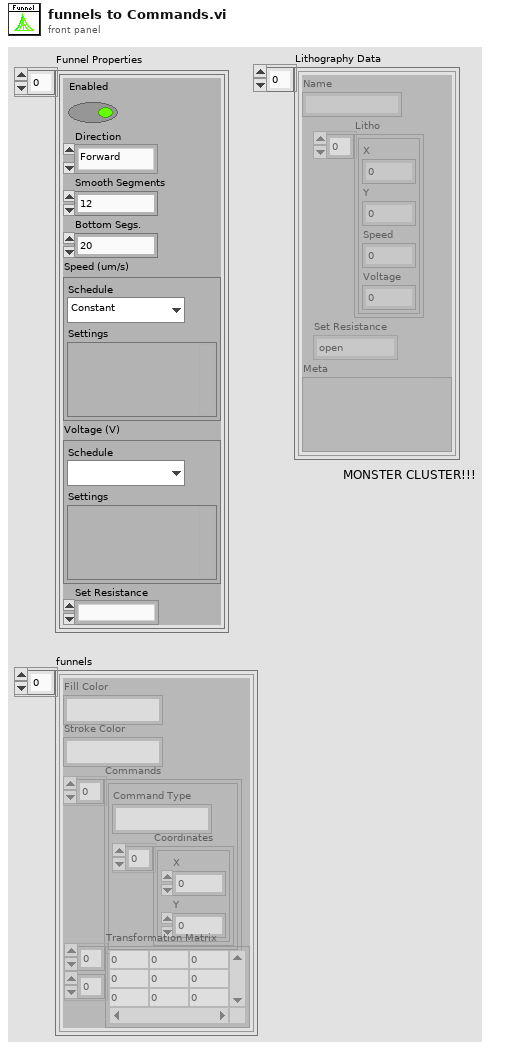
[diagram p1: front panel]
types:
  T1 = typedef "Relay-Box.lvclass/Resistor--enum.ctl" = enum16{"open", "discharge tip", "0 ohms", "100k ohm", "10M ohm", "1G ohm"}
  T2 = cluster{"Name":string, "Litho":cluster{"X":dbl, "Y":dbl, "Speed":dbl, "Voltage":dbl}[], "Set Resistance":T1, "Meta":variant}[]
  T3 = typedef "Funnel Properties - cluster.ctl" = cluster{"Enabled":bool, "Direction":u16, "Smooth Segments":dbl, "Bottom Segs.":dbl, "Speed (um/s)":T4, "Voltage (V)":T4, "Set Resistance":T1}
  T4 = typedef "Voltage - cluster.ctl" = cluster{"Schedule":T5, "Settings":variant}
  T5 = typedef "Schedule - enum.ctl" = enum16{"Constant", "Ramp", "Fn. Generator", "Formula"}
  T6 = typedef "NI_Matrix.lvlib/RealMatrix.ctl" = dbl[][]
  T7 = cluster{"Fill Color":string, "Stroke Color":string, "Commands":cluster{"Command Type":string, "Coordinates":cluster{"X":dbl, "Y":dbl}[]}[], "Transformation Matrix":T6}[]
  T8 = cluster{"Name":string, "Litho":cluster{"X":dbl, "Y":dbl, "Speed":dbl, "Voltage":dbl}[], "Set Resistance":T1, "Meta":variant}
  T9 = cluster{"Command Type":string, "Coordinates":cluster{"X":dbl, "Y":dbl}[]}[]
  T10 = cluster{string, "Funnel Path":cluster{dbl, dbl}[]}
  T11 = cluster{"Name":string, "Litho":cluster{"X":dbl, "Y":dbl, "Speed":dbl, "Voltage":dbl}[], "Set Resistance":T1}
  T12 = cluster{"X":dbl, "Y":dbl, "Speed":dbl, "Voltage":dbl}[]
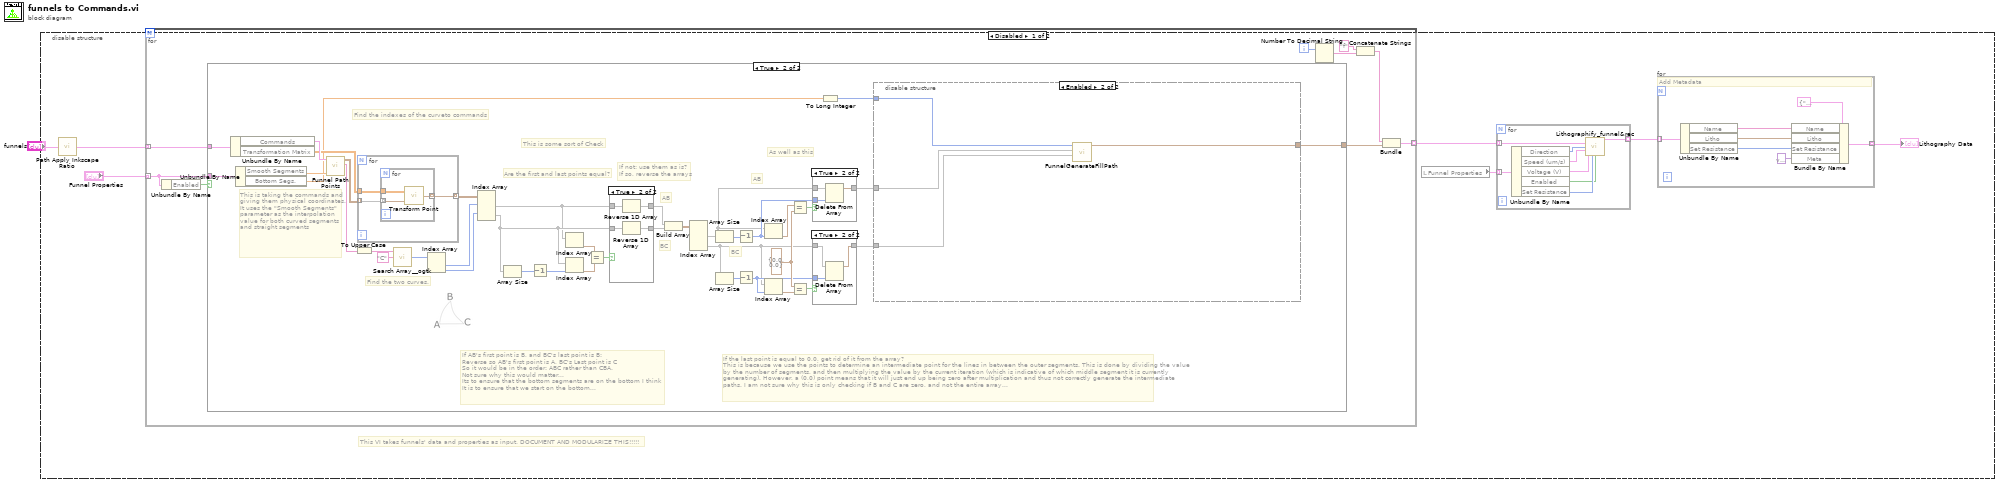
[diagram p0: block diagram]
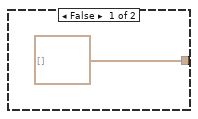
[diagram p2: hidden frame]
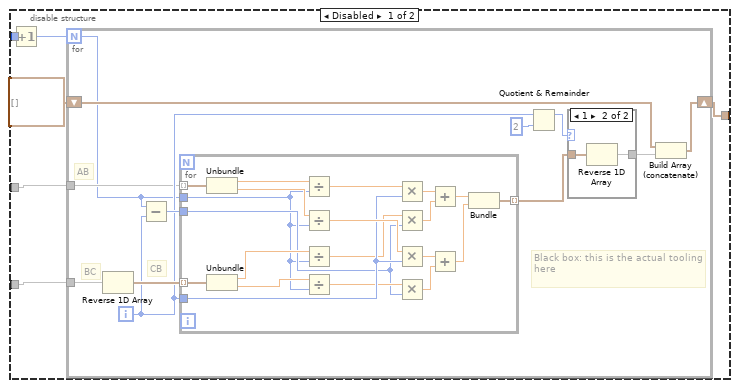
[diagram p3: hidden frame]
diagram:
  n1 = disable-structure shown="Disabled" {
    frame Disabled {
      # "This VI takes funnels' data and properties as input. DOCUMENT AND MODULARIZE THIS!!!!!"
      n2 = call "Path Apply Inkscape Ratio.vi"("paths in"="funnels") -> ("paths out"=w6:T7)
      n3 = for {
        tunnel: w6 -> [w31] mode=indexing
        tunnel: "Funnel Properties" -> [w25] mode=indexing
        tunnel: [w29] -> w3 mode=indexing
        i -> [w26]
        n4 = Unbundle By Name(w25) -> ("Enabled"=w24:bool)
        n5 = case shown="True" w24 {
          tunnel: w25 -> [_ w71]
          tunnel: w31 -> [_ w70]
          tunnel: [cluster{dbl, dbl}[] [] w50] -> w23
          frame False {
          }
          frame True {
            w61 = cluster{"X":dbl, "Y":dbl} {"X"=0.0, "Y"=0.0} ("y")
            # "BC"
            # "AB"
            # "BC"
            # "AB"
            # "Find the two curves."
            # "This is taking the commands and giving them physical coordinates. It uses the \"Smooth Segments\" parameter as the interpolation value for both curved segments and straight segments"
            # "As well as this"
            # "This is some sort of Check"
            # "If the last point is equal to 0,0, get rid of it from the array?\nThis is because we use the points to determine an intermediate point for the lines in between the outer segments. This is done by dividing the value by the number of segments, and then multiplying the value by the current iteration (which is indicative of which middle segment it is currently generating). However, a (0,0) point means that it will just end up being zero after multiplication and thus not correctly generate the intermediate paths. I am not sure why this is only checking if B and C are zero, and not the entire array..."
            # "If AB's first point is B, and BC's last point is B:\nReverse so AB's first point is A, BC's Last point is C\nSo it would be in the order: ABC rather than CBA.\nNot sure why this would matter...\nIts to ensure that the bottom segments are on the bottom I think\nIt is to ensure that we start on the bottom..."
            # "Find the indexes of the curveto commands"
            # "If not: use them as is?\nIf so, reverse the arrays"
            # "Are the first and last points equal?"
            n6 = Unbundle By Name(w70) -> ("Commands"=w51:T9, "Transformation Matrix"=w48:T6)
            n7 = Unbundle By Name(w71) -> ("Smooth Segments"=w52:dbl, "Bottom Segs."=w38:dbl)
            n8 = call "Funnel Path Points.vi"("Smooth Segments"=w52, "Commands"=w51) -> ("Commands"=w43:string[], "Array"=w45:cluster{"X":dbl, "Y":dbl}[][])  [unwired: 7 in, 1 out]
            n9 = To Upper Case(1:w43) -> (0:w42:string[])
            n10 = for {
              tunnel: w45 -> [w119] mode=indexing
              tunnel: [w118] -> w49 mode=indexing
              tunnel: w48 -> [w117]
              n11 = for {
                tunnel: w119 -> [w122] mode=indexing
                tunnel: [w121] -> w118 mode=indexing
                tunnel: w117 -> [w120]
                n12 = call "Transform Point.vi"("Point to Transform"=w122, "Transformation Matrix"=w120) -> ("Transformed Point"=w121:cluster{"X":dbl, "Y":dbl})
              }
            }
            n13 = call-poly <userlib>:"Search Array__ogtk.vi"("Array"=w42, "Element Data"="C") -> ("Indices of Elements"=w41:i32[])  [unwired: 7 in]
            n14 = Index Array(array=w41) -> (element #1=w40:i32, element #2=w39:i32)  [unwired: 2 in]
            n15 = Index Array(array=w49, index (row) #1=w40, index (row) #2=w39) -> (element #1=w46:cluster{"X":dbl, "Y":dbl}[], element #2=w47:cluster{"X":dbl, "Y":dbl}[])  [unwired: 2 in]
            n16 = Array Size(array=w47) -> (size(s)=w68:i32)
            n17 = Decrement(x=w68) -> (x-1=w67:i32)
            n18 = Index Array(array=w46) -> (element=w36:cluster{"X":dbl, "Y":dbl})  [unwired: 1 in]
            n19 = Index Array(array=w47, index=w67) -> (element=w37:cluster{"X":dbl, "Y":dbl})
            n20 = Equal?(x=w36, y=w37) -> (x = y?=w66:bool)
            n21 = case shown="True" w66 {
              tunnel: w46 -> [w132 w136]
              tunnel: w47 -> [w131 w135]
              tunnel: [w132 w134] -> w65
              tunnel: [w131 w133] -> w64
              frame False {
              }
              frame True {
                n22 = Reverse 1D Array(array=w136) -> (reversed array=w134:cluster{"X":dbl, "Y":dbl}[])
                n23 = Reverse 1D Array(array=w135) -> (reversed array=w133:cluster{"X":dbl, "Y":dbl}[])
              }
            }
            n24 = Build Array(w65, w64) -> (w69:cluster{"X":dbl, "Y":dbl}[][])
            n25 = Index Array(array=w69) -> (element #1=w33:cluster{"X":dbl, "Y":dbl}[], element #2=w34:cluster{"X":dbl, "Y":dbl}[])  [unwired: 4 in]
            n26 = Array Size(array=w33) -> (size(s)=w59:i32)
            n27 = Array Size(array=w34) -> (size(s)=w60:i32)
            n28 = Decrement(x=w59) -> (x-1=w58:i32)
            n29 = Decrement(x=w60) -> (x-1=w55:i32)
            n30 = Index Array(array=w33, index=w58) -> (element=w63:cluster{"X":dbl, "Y":dbl})
            n31 = Index Array(array=w34, index=w55) -> (element=w62:cluster{"X":dbl, "Y":dbl})
            n32 = Equal?(x=w63, y=w61) -> (x = y?=w56:bool)
            n33 = Equal?(x=w61, y=w62) -> (x = y?=w53:bool)
            n34 = case shown="True" w56 {
              tunnel: w33 -> [w127 w130]
              tunnel: w58 -> [_ w128]
              tunnel: [w127 w129] -> w57
              frame False {
              }
              frame True {
                n35 = Delete From Array(array=w130, index=w128) -> (array with subset deleted=w129:cluster{"X":dbl, "Y":dbl}[])  [unwired: 1 in, 1 out]
              }
            }
            n36 = case shown="True" w53 {
              tunnel: w34 -> [w123 w126]
              tunnel: w55 -> [_ w124]
              tunnel: [w123 w125] -> w54
              frame False {
              }
              frame True {
                n37 = Delete From Array(array=w126, index=w124) -> (array with subset deleted=w125:cluster{"X":dbl, "Y":dbl}[])  [unwired: 1 in, 1 out]
              }
            }
            n38 = To Long Integer(number=w38) -> (32bit integer=w35:i32)
            n39 = disable-structure shown="Enabled" {
              disable-tunnel: w57 -> [w76 w115]
              disable-tunnel: w54 -> [w75 w114]
              disable-tunnel: [w74 w116] -> w50
              disable-tunnel: w35 -> [w73 w113]
              frame Disabled {
                n40 = Increment(x=w73) -> (x+1=w72:i32)
                n41 = for {
                  N: w72 -> [w79]
                  tunnel: w75 -> [w81]
                  shift-right: [w78] -> w74
                  shift-left: cluster{dbl, dbl}[] [] -> [w88]
                  tunnel: w76 -> [w80]
                  i -> [w86]
                  # "CB"
                  # "BC"
                  # "AB"
                  # "Black box: this is the actual tooling here"
                  n42 = Reverse 1D Array(array=w81) -> (reversed array=w87:cluster{"X":dbl, "Y":dbl}[])
                  n43 = Subtract(x=w79, y=w86) -> (x-y=w89:i32)
                  n44 = for {
                    tunnel: w80 -> [w112] mode=indexing
                    tunnel: w87 -> [w111] mode=indexing
                    tunnel: w86 -> [w106]
                    tunnel: w89 -> [w101]
                    tunnel: [w95] -> w83 mode=indexing
                    tunnel: w79 -> [w94]
                    n45 = Unbundle(w112) -> ("X"=w110:dbl, "Y"=w108:dbl)
                    n46 = Unbundle(w111) -> ("X"=w105:dbl, "Y"=w104:dbl)
                    n47 = Divide(x=w110, y=w94) -> (x/y=w109:dbl)
                    n48 = Divide(x=w108, y=w94) -> (x/y=w107:dbl)
                    n49 = Divide(x=w105, y=w94) -> (x/y=w103:dbl)
                    n50 = Divide(x=w104, y=w94) -> (x/y=w102:dbl)
                    n51 = Multiply(x=w109, y=w106) -> (x*y=w100:dbl)
                    n52 = Multiply(x=w103, y=w101) -> (x*y=w99:dbl)
                    n53 = Multiply(x=w107, y=w106) -> (x*y=w98:dbl)
                    n54 = Multiply(x=w102, y=w101) -> (x*y=w97:dbl)
                    n55 = Add(x=w100, y=w99) -> (x+y=w96:dbl)
                    n56 = Add(x=w98, y=w97) -> (x+y=w93:dbl)
                    n57 = Bundle(w96, w93) -> (w95:cluster{dbl, dbl})  [unwired: 1 in]
                  }
                  n58 = Quotient & Remainder(x=w86, y=2) -> (x-y*floor(x/y)=w84:i32)  [unwired: 1 out]
                  n59 = case shown="1" w84 {
                    tunnel: w83 -> [w90 w92]
                    tunnel: [w90 w91] -> w82
                    frame 0, Default {
                    }
                    frame 1 {
                      n60 = Reverse 1D Array(array=w92) -> (reversed array=w91:cluster{dbl, dbl}[])
                    }
                  }
                  n61 = Build Array (concatenate)(w88, w82) -> (w78:cluster{dbl, dbl}[])
                }
              }
              frame Enabled {
                n62 = call "FunnelGenerateFillPath.vi"("Curve 2"=w114, "Curve 1"=w115, "Bottom Segments"=w113) -> ("Funnel Path"=w116:cluster{dbl, dbl}[])  [unwired: 8 in]
              }
            }
          }
        }
        n63 = Number To Decimal String(number=w26) -> (decimal integer string=w27:string)  [unwired: 1 in]
        n64 = Concatenate Strings("f" ("string"), w27) -> (w30:string)
        n65 = Bundle(w30, "Funnel Path"=w23) -> (w29:T10)  [unwired: 1 in]
      }
      n66 = local read "Funnel Properties"() -> (w4:T3[])
      n67 = for {
        tunnel: w4 -> [w22] mode=indexing
        tunnel: w3 -> [w20] mode=indexing
        tunnel: [w19] -> w2 mode=indexing
        n68 = Unbundle By Name(w22) -> ("Direction"=w18:u16, "Speed (um/s)"=w21:T4, "Voltage (V)"=w15:T4, "Enabled"=w16:bool, "Set Resistance"=w17:T1)
        n69 = call "Lithographify_funnel&rec.vi"("Data In"=w20, "Direction"=w18, "Speed (µm/s)"=w21, "Voltage (V)"=w15, "Set Resistance"=w17, "Enabled"=w16) -> ("Lithography Data"=w19:T11)  [unwired: 9 in]
      }
      n70 = for {
        tunnel: w2 -> [w14] mode=indexing
        tunnel: [w8] -> w1 mode=indexing
        # "Add Metadata"
        n71 = Unbundle By Name(w14) -> ("Name"=w12:string, "Litho"=w11:T12, "Set Resistance"=w10:T1)
        n72 = Bundle By Name(cluster=T8 {"Name"="", "Litho"=[], "Set Resistance"=enum."open", "Meta"=variant} ("Pattern Data"), "Name"=w12, "Litho"=w11, "Set Resistance"=w10, "Meta"=variant) -> (w8:T8)
      }
      "Lithography Data" <- w1
    }
    frame Enabled {
    }
  }
